vi "Create.vi"(8 "Error In":errorcluster, 11 "reference in":refnum<class "Flir A700.lvclass">) -> (0 "Error Out":errorcluster, 3 "reference out":refnum<class "Flir A700.lvclass">)   [LabVIEW 2024, in "Flir A700.lvclass"]
uses:
  Flir A700.lvclass
  Flir A700.lvclass/Flir A700.ctl
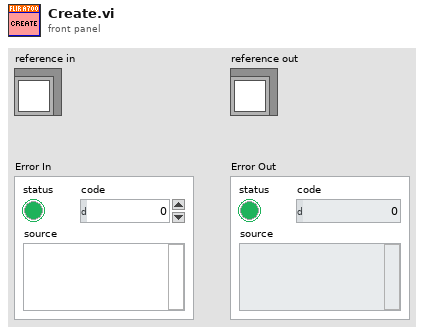
[diagram p1: front panel]
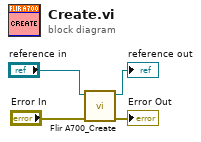
[diagram p0: block diagram]
diagram:
  n1 = call "Flir A700_Create.vi"("Error In"="Error In", "reference in"="reference in") -> ("Error Out"=→"Error Out":errorcluster, "reference out"=→"reference out":refnum<class "Flir A700.lvclass">)  [unwired: 8 in]
